vi "airconditioner.vi"() -> ()   [LabVIEW 2026]
uses:
  <vilib>/numeric/Random Number (Range) DBL.vi
panel:
  out "Current Room Temperature":dbl(slide) scale=0.0..50.0
  in  "Confirm":bool
  in  "Target Temperature":dbl(slide) scale=0.0..50.0
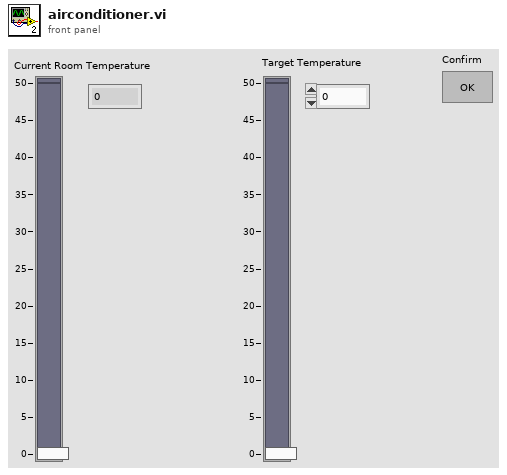
[diagram p1: front panel]
types:
  T1 = enum16{"Init", "Select Temperature", "Temperature Monitoring", "Cool", "Heat", "Exit"}
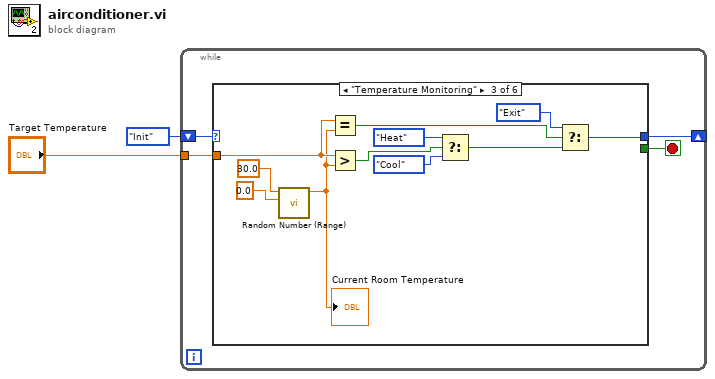
[diagram p0: block diagram]
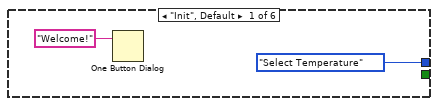
[diagram p2: hidden frame]
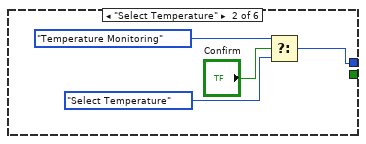
[diagram p3: hidden frame]
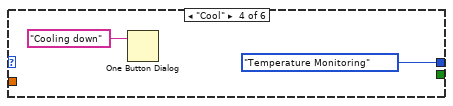
[diagram p4: hidden frame]
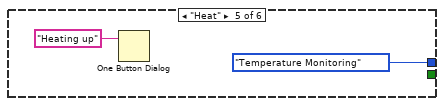
[diagram p5: hidden frame]
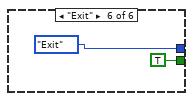
[diagram p6: hidden frame]
diagram:
  n1 = while {
    shift-right: [w5] -> _
    shift-left: T1."Init" -> [w6]
    tunnel: "Target Temperature" -> [w4]
    stop <- w3 stop-if-true
    n2 = case shown="\"Temperature Monitoring\"" w6 {
      tunnel: [T1."Select Temperature" w10 w19 T1."Temperature Monitoring" T1."Temperature Monitoring" T1."Exit"] -> w5
      tunnel: w4 -> [_ _ w16 _ _ _]
      tunnel: [_ _ _ _ _ TRUE] -> w3
      frame "Init", Default {
        n3 = One Button Dialog(message="Welcome!") -> ()  [unwired: 1 in, 1 out]
      }
      frame "Select Temperature" {
        n4 = Select(t=T1."Temperature Monitoring", s="Confirm", f=T1."Select Temperature") -> (s? t:f=w10:T1)
      }
      frame "Temperature Monitoring" {
        n5 = call-poly <vilib>:"Random Number (Range).vi"("lower bound (0)"=0.0, "upper bound (100)"=30.0) -> ("number"=w13:dbl)  [unwired: 9 in]
        "Current Room Temperature" <- w13
        n6 = Equal?(x=w16, y=w13) -> (x = y?=w20:bool)
        n7 = Greater?(x=w16, y=w13) -> (0:w22:bool)
        n8 = Select(t=T1."Heat", s=w22, f=T1."Cool") -> (s? t:f=w18:T1)
        n9 = Select(t=T1."Exit", s=w20, f=w18) -> (s? t:f=w19:T1)
      }
      frame "Cool" {
        n10 = One Button Dialog(message="Cooling down") -> ()  [unwired: 1 in, 1 out]
      }
      frame "Heat" {
        n11 = One Button Dialog(message="Heating up") -> ()  [unwired: 1 in, 1 out]
      }
      frame "Exit" {
      }
    }
  }
